vi "Loop_PCM_SEN.vi"() -> ()   [LabVIEW 2017, in "System_Status.lvlib"]
uses:
  System_Status.lvlib
  TypeDef Share All/CLUSTER_PCM_Status.ctl
  CLUSTER_System_CMD.ctl
  Global Share All/Global_STOP.vi
  Global_CMD.vi
  Global_SEN Write_Data.vi
panel:
  out "Cycle Time (S)":dbl format="%.3g"
  in  "Target Time(ms)":u32=50
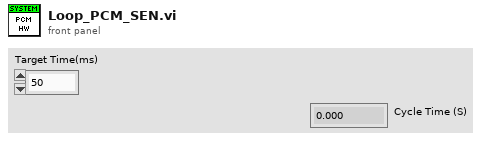
[diagram p1: front panel]
types:
  T1 = typedef "System_Status.lvlib/CLUSTER_System_CMD.ctl" = cluster{"Enable PCM Monitoring":bool, "Enable PDP Monitoring":bool, "Enable RoboRio Monitoring":bool}
  T2 = typedef "CLUSTER_PCM_Status.ctl" = cluster{"Current (A)":dbl, "All Solenoid Faults":bool[], "Input Voltage":dbl, "Solenoid Voltage":dbl, "Comp. Fault":bool}
  T3 = cluster{"PCM ID":i32, "Target Time(ms)":u32, "Current Time":timestamp, "Previous Time":timestamp, "Cycle Time (S)":dbl, "PCM Status":T2, "Enabled":T1}
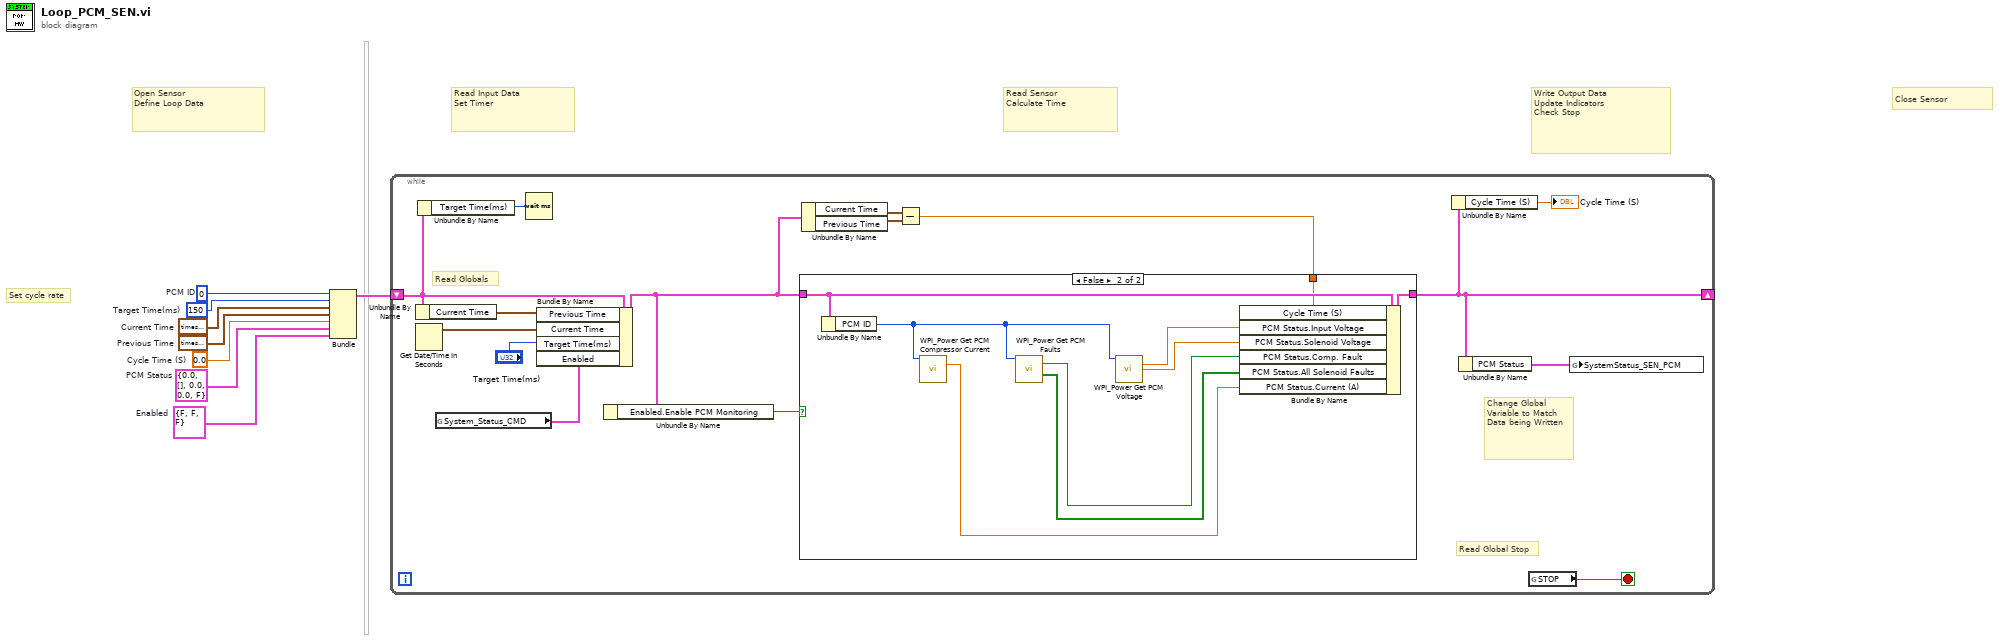
[diagram p0: block diagram]
diagram:
  w1 = T1 {"Enable PCM Monitoring"=FALSE, "Enable PDP Monitoring"=FALSE, "Enable RoboRio Monitoring"=FALSE}  # Enabled
  w2 = T2 {"Current (A)"=0.0, "All Solenoid Faults"=[], "Input Voltage"=0.0, "Solenoid Voltage"=0.0, "Comp. Fault"=FALSE}  # PCM Status
  w3 = 0  # PCM ID
  w4 = 0.0  # Cycle Time (S)
  w8 = timestamp(0 s since 1904-01-01)  # Previous Time
  w7 = timestamp(0 s since 1904-01-01)  # Current Time
  w6 = u32 150  # Target Time(ms)
  # "Close Sensor"
  # "Write Output Data\nUpdate Indicators\nCheck Stop"
  # "Read Sensor\nCalculate Time"
  # "Read Input Data\nSet Timer"
  # "Open Sensor\nDefine Loop Data"
  # "Set cycle rate"
  n1 = Bundle("PCM ID"=w3, "Target Time(ms)"=w6, "Current Time"=w7, "Previous Time"=w8, "Cycle Time (S)"=w4, "PCM Status"=w2, "Enabled"=w1) -> (w5:T3)  [unwired: 1 in]
  n2 = while {
    shift-right: [w14] -> _
    shift-left: w5 -> [w16]
    stop <- w23 stop-if-true
    # "Change Global\nVariable to Match\nData being Written"
    # "Read Globals"
    # "Read Global Stop"
    n3 = Unbundle By Name(w16) -> ("Current Time"=w20:timestamp)
    n4 = Get Date/Time In Seconds() -> (seconds since 1Jan1904=w21:timestamp)
    n5 = Unbundle By Name(w16) -> ("Target Time(ms)"=w15:u32)
    n6 = global read "Global_CMD.vi" "System_Status_CMD"() -> (w11:T1)
    n7 = Wait (ms)(milliseconds to wait=w15) -> ()  [unwired: 1 out]
    n8 = Bundle By Name(cluster=w16, "Previous Time"=w20, "Current Time"=w21, "Target Time(ms)"="Target Time(ms)", "Enabled"=w11) -> (w10:T3)
    n9 = Unbundle By Name(w10) -> ("Enabled.Enable PCM Monitoring"=w9:bool)
    n10 = Unbundle By Name(w10) -> ("Current Time"=w19:timestamp, "Previous Time"=w18:timestamp)
    n11 = Subtract(x=w19, y=w18) -> (x-y=w12:dbl)
    n12 = case shown="False" w9 {
      tunnel: w10 -> [w24 w33]
      tunnel: [w24 w32] -> w14
      tunnel: w12 -> [_ w31]
      frame True {
      }
      frame False {
        n13 = Unbundle By Name(w33) -> ("PCM ID"=w30:i32)
        n14 = call <vilib>:"WPI_Power Get PCM Compressor Current.vi"("Pneumatics Control Module (0)"=w30) -> ("current (A)"=w29:dbl)  [unwired: 13 in, 1 out]
        n15 = call <vilib>:"WPI_Power Get PCM Faults.vi"("Pneumatics Control Module (0)"=w30) -> ("Compressor Fault"=w26:bool, "All Solenoid Faults"=w28:bool[])  [unwired: 11 in, 2 out]
        n16 = call <vilib>:"WPI_Power Get PCM Voltage.vi"("Pneumatics Control Module (0)"=w30) -> ("Input Voltage"=w25:dbl, "Solenoid Voltage"=w27:dbl)  [unwired: 12 in, 1 out]
        n17 = Bundle By Name(cluster=w33, "Cycle Time (S)"=w31, "PCM Status.Input Voltage"=w25, "PCM Status.Solenoid Voltage"=w27, "PCM Status.Comp. Fault"=w26, "PCM Status.All Solenoid Faults"=w28, "PCM Status.Current (A)"=w29) -> (w32:T3)
      }
    }
    n18 = Unbundle By Name(w14) -> ("Cycle Time (S)"=→"Cycle Time (S)":dbl)
    n19 = Unbundle By Name(w14) -> ("PCM Status"=w22:T2)
    n20 = global read "Global_STOP.vi" "STOP"() -> (w23:bool)
    n21 = global write "Global_SEN Write_Data.vi" "SystemStatus_SEN_PCM"(w22) -> ()
  }
